vi "Restart APAR Motion Loop.vi"(7 "Motion restart":enum16{"NoOp", "Start", "Stop"}(ring)=enum."Start", 8 "error in":errorcluster, 11 "MessageQues":T1) -> (0 "error out":errorcluster)   [LabVIEW 2018]
uses:
  Support/MessageQue/VXM Main Test App/MultipleMessageQues vxm.ctl
  Support/MessageQue/MessageQue.ctl
  Support/MessageQue/MessageCluster.ctl
  Support/MessageQue/MessageQue.lvlib
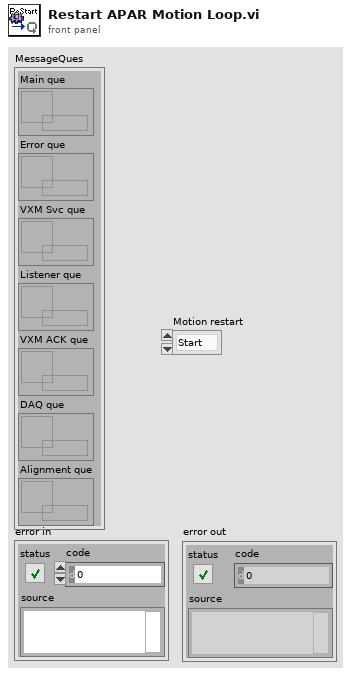
[diagram p1: front panel]
types:
  T1 = typedef "MultipleMessageQues vxm.ctl" = cluster{"Main que":T2, "Error que":T2, "VXM Svc que":T2, "Listener que":T2, "VXM ACK que":T2, "DAQ que":T2, "Alignment que":T2}
  T2 = typedef "MessageQue.lvlib/MessageQue.ctl" = refnum<queue>
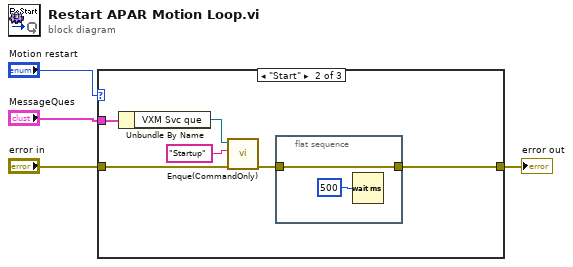
[diagram p0: block diagram]
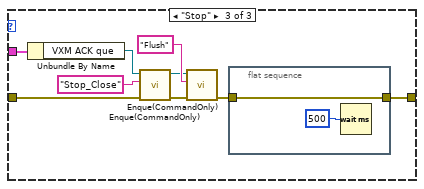
[diagram p3: hidden frame]
diagram:
  n1 = case shown="\"Start\"" "Motion restart" {
    tunnel: "MessageQues" -> [_ w10 w21]
    tunnel: "error in" -> [w5 w8 w19]
    tunnel: [w5 w6 w18] -> w2
    frame "NoOp", Default {
    }
    frame "Start" {
      n2 = Unbundle By Name(w10) -> ("VXM Svc que"=w9:T2)
      n3 = call "Enque(CommandOnly).vi"("error in"=w8, "Message Command"="Startup", "Message que"=w9) -> ("error out"=w7:errorcluster)  [unwired: 7 in, 1 out]
      n4 = flat-sequence {
        tunnel: w7 -> [w12]
        tunnel: [w12] -> w6
        frame #0 {
          n5 = Wait (ms)(milliseconds to wait=u32 500) -> ()  [unwired: 1 out]
        }
      }
    }
    frame "Stop" {
      n6 = Unbundle By Name(w21) -> ("VXM ACK que"=w20:T2)
      n7 = call "Enque(CommandOnly).vi"("error in"=w19, "Message Command"="Stop_Close", "Message que"=w20) -> ("error out"=w15:errorcluster, "Message que out"=w16:T2)  [unwired: 7 in]
      n8 = call "Enque(CommandOnly).vi"("error in"=w15, "Message Command"="Flush", "Message que"=w16) -> ("error out"=w14:errorcluster)  [unwired: 7 in, 1 out]
      n9 = flat-sequence {
        tunnel: w14 -> [w23]
        tunnel: [w23] -> w18
        frame #0 {
          n10 = Wait (ms)(milliseconds to wait=u32 500) -> ()  [unwired: 1 out]
        }
      }
    }
  }
  "error out" <- w2
